vi "CANOpen Debug print.vi"(8 "error in (no error)":errorcluster, 11 "ID":u8) -> ()   [LabVIEW 2013, in "CANOpen Addon Custom Device.lvlib"]
uses:
  CANOpen Addon Custom Device.lvlib
  <vilib>/NI Veristand/Custom Device Tools/Custom Device Utility Library/Custom Device Utility Library.lvlib
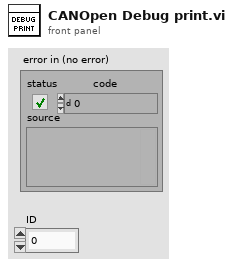
[diagram p1: front panel]
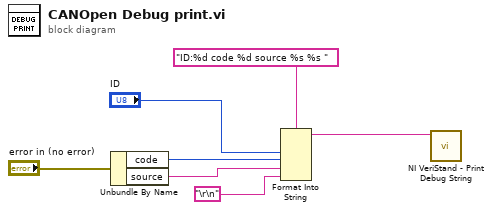
[diagram p0: block diagram]
diagram:
  n1 = Unbundle By Name("error in (no error)") -> ("code"=w4:i32, "source"=w3:string)
  n2 = Format Into String(format string="ID:%d code %d source %s %s ", "ID", w4, w3, "\r\n") -> (resulting string=w1:string)  [unwired: 2 in, 1 out]
  n3 = call <vilib>:"NI VeriStand - Print Debug String.vi"("Message"=w1) -> ()  [unwired: 10 in, 1 out]
